vi "AB_Log_ClassData.vi"(8 "error in (no error)":errorcluster, 10 "sectionName":string, 11 "AB_Build.lvclass":refnum<class "AB_Build.lvclass">) -> (0 "error out":errorcluster)   [LabVIEW 2020]
uses:
  <vilib>/AppBuilder/AB_Classes/Build/AB_Build.lvclass
  <vilib>/AppBuilder/AB_Classes/Source/AB_Source.lvclass
  <vilib>/AppBuilder/AB_Classes/Destination/AB_Destination.lvclass
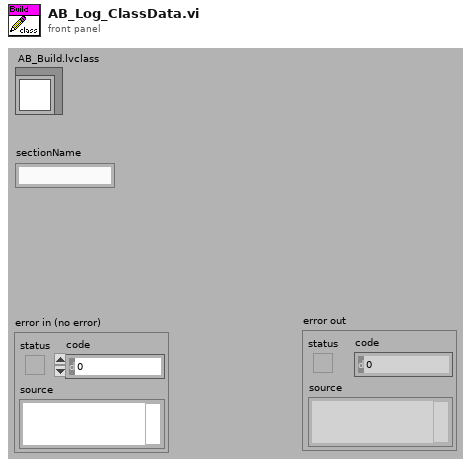
[diagram p1: front panel]
types:
  T1 = typedef "AB_Build.ctl" = cluster{"buildSpecName":string, "buildSpecDescription":string, "destinations":refnum<class "AB_Destination.lvclass">[], "exclusionOption":T2, "defaultLanguage":string, "supportedLanguages":string[], "excludedDirectories":path[], "buildContext":refnum<vi>, "buildObject":T3, "preview":bool, "programatic":bool, "progressBarEvents":T4, "userLog_Path":path, "preActionID":string, "preAction_Path":path, "postActionID":string, "postAction_Path":path, "eng_checkForBrokenVIs?":bool, "eng_verboseLinkerErrors?":bool, "localDest_Path":path, "targetDest_Path":path, "removeVIObject":u16, "cache":refnum<class "PreviewCache.lvclass">, "use cache":bool, "previewCache_ID":string, "buildCache_ID":string, "eng_TempLocalDest_Path":path, "eng_collectDependencies?":bool, "versionInfo":cluster{"buildVersion":cluster{"major":u16, "minor":u16, "patch":u16, "build":u16}, "autoIncrement":bool}, "eng_enableVIChecksums":bool}
  T2 = typedef "AB_Exclusion_Option.ctl" = cluster{"typedefs":bool, "polymorphicVIs":bool, "unusedLibraryItems":bool, "modifyLibraryFile":bool, "edit-timeDependencies":bool, "inlineVIs":bool, "dependent PPLs":bool, "dependent DLLs":bool}
  T3 = typedef "ItemRef.ctl" = u64
  T4 = typedef "provcom_ProgressBar_Events.ctl" = cluster{"newJob":refnum<user-event>, "newItem":refnum<user-event>, "errorMsg":T5, "cancel":refnum<user-event>}
  T5 = typedef "mxLvBuildError.ctl" = refnum<user-event>
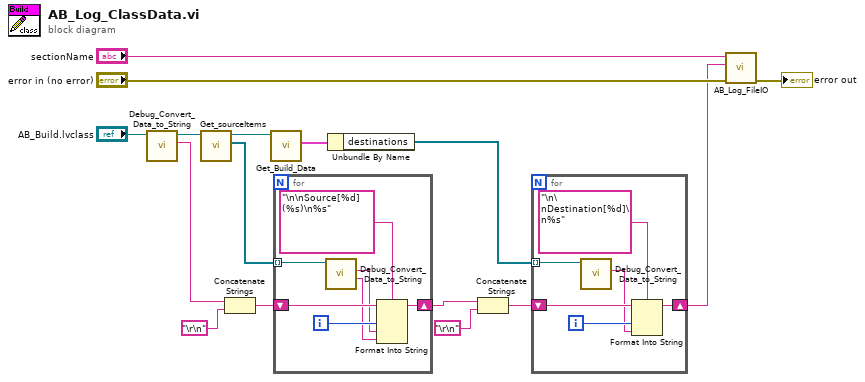
[diagram p0: block diagram]
diagram:
  n1 = call-dynamic "Debug_Convert_Data_to_String.vi"("AB_Build in"="AB_Build.lvclass") -> ("classData"=w11:string, "AB_Build out"=w13:refnum<class "AB_Build.lvclass">)  [unwired: 8 in, 1 out]
  n2 = call <vilib>:"Get_sourceItems.vi"("Class in"=w13) -> ("sourceItems"=w9:refnum<class "AB_Source.lvclass">[], "Class out"=w2:refnum<class "AB_Build.lvclass">)  [unwired: 8 in, 1 out]
  n3 = Concatenate Strings(w11, "\r\n") -> (w10:string)
  n4 = call <vilib>:"Get_Build_Data.vi"("Class in"=w2) -> ("data"=w3:T1)  [unwired: 8 in, 2 out]
  n5 = for {
    shift-right: [w21] -> w6
    shift-left: w10 -> [w22]
    tunnel: w9 -> [w18] mode=indexing
    i -> [w20]
    n6 = call-dynamic "Debug_Convert_Data_to_String.vi"("AB_Source in"=w18) -> ("classData"=w17:string, "sourceType"=w19:string)  [unwired: 7 in, 2 out]
    n7 = Format Into String(format string="\n\nSource[%d] (%s)\n%s", initial string=w22, w20, w19, w17) -> (resulting string=w21:string)  [unwired: 1 in, 1 out]
  }
  n8 = Unbundle By Name(w3) -> ("destinations"=w1:refnum<class "AB_Destination.lvclass">[])
  n9 = Concatenate Strings(w6, "\r\n") -> (w8:string)
  n10 = for {
    shift-right: [w27] -> w5
    shift-left: w8 -> [w28]
    tunnel: w1 -> [w25] mode=indexing
    i -> [w26]
    n11 = call-dynamic "Debug_Convert_Data_to_String.vi"("AB_Destination in"=w25) -> ("classData"=w24:string)  [unwired: 8 in, 2 out]
    n12 = Format Into String(format string="\n\nDestination[%d]\n%s", initial string=w28, w26, w24) -> (resulting string=w27:string)  [unwired: 1 in, 1 out]
  }
  n13 = call <vilib>:"AB_Log_FileIO.vi"("error in (no error)"="error in (no error)", "data"=w5, "newSection"="sectionName") -> ("error out"=→"error out":errorcluster)  [unwired: 8 in]
